vi "Check Device Out.vi"(8 "error in (no error)":errorcluster, 10 "Device GUID":string, 11 "Controller in":refnum<class "Controller.lvclass">) -> (0 "error out":errorcluster, 3 "Controller out":refnum<class "Controller.lvclass">)   [LabVIEW 2016, in "Controller Actor.lvlib" / "Controller.lvclass"]
uses:
  <userlib>/Common Components/Controller/Controller.lvclass
  <userlib>/Common Components/Controller UI/Update DT event data.ctl
  <userlib>/Common Components/Controller UI/Update DT Cmd.ctl
  <userlib>/Common Components/Controller UI/Update DT event data - checked out.ctl
  <userlib>/Common Components/Controller UI Messages/Update DT Event Msg/Update DT Event Msg.lvclass/Update DT Event Msg.ctl
  <vilib>/ActorFramework/Message Enqueuer/Message Enqueuer.lvclass/Message Enqueuer.ctl
  <vilib>/ActorFramework/Message Enqueuer/Enqueue.vi
  <userlib>/Common Components/Controller UI Messages/Update DT Event Msg/Update DT Event Msg.lvclass
  C:/Program Files (x86)/National Instruments/LabVIEW 2016/vi.lib/ActorFramework/Message/Message.lvclass
  <vilib>/ActorFramework/Message Priority Queue/Priority Enqueue.vi
  <userlib>/Common Components/Controller UI/Controller UI.lvclass
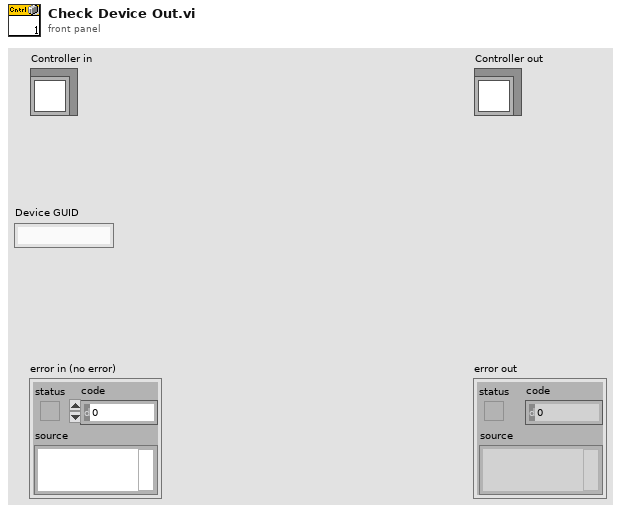
[diagram p1: front panel]
types:
  T1 = typedef "Controller UI.lvlib/Controller UI.lvclass/Update DT event data - checked out.ctl" = cluster{"GUID":string, "checked-out?":bool}
  T2 = typedef "Controller UI.lvlib/Controller UI.lvclass/Update DT event data.ctl" = cluster{"Cmd":T3, "Data Array":variant[]}
  T3 = typedef "Controller UI.lvlib/Controller UI.lvclass/Update DT Cmd.ctl" = enum16{"Update HWtype\\HWplugin array", "Update Checked-out", "Update COMM Status", "Load DevInfo from File", "Save DevInfo to File", "Update COMM Address List"}
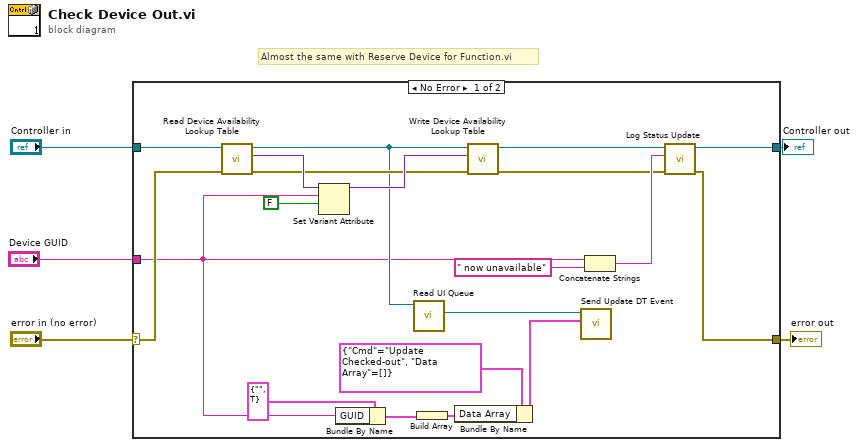
[diagram p0: block diagram]
diagram:
  # "Almost the same with Reserve Device for Function.vi"
  n1 = case shown="No Error" "error in (no error)" {
    selector: "error in (no error)" -> [w16 w27]
    tunnel: [w15 w27] -> w4
    tunnel: [w19 w26] -> w2
    tunnel: "Controller in" -> [w25 w26]
    tunnel: "Device GUID" -> [w10 _]
    frame No Error {
      n2 = call <userlib>:"Read Device Availability Lookup Table.vi"("error in (no error)"=w16, "Controller in"=w25) -> ("error out"=w18:errorcluster, "Device Availability Lookup Table"=w24:variant, "Controller out"=w14:refnum<class "Controller.lvclass">)  [unwired: 7 in]
      n3 = Set Variant Attribute(Variant=w24, name=w10, value=FALSE) -> (Variant out=w23:variant)  [unwired: 1 in, 2 out]
      n4 = Bundle By Name(cluster=T1 {"GUID"="", "checked-out?"=TRUE} ("Cluster"), "GUID"=w10) -> (w8:T1)
      n5 = call <userlib>:"Read UI Queue.vi"("UI Controller in"=w14) -> ("UI Queue"=w13:refnum<class "Message Enqueuer.lvclass">)  [unwired: 8 in, 2 out]
      n6 = Build Array(w8) -> (w7:T1[])
      n7 = Bundle By Name(cluster=T2 {"Cmd"=enum."Update Checked-out", "Data Array"=[]} ("event data"), "Data Array"=w7) -> (w11:T2)
      n8 = call <userlib>:"Write Device Availability Lookup Table.vi"("error in (no error)"=w18, "Device Availability Lookup Table"=w23, "Controller in"=w14) -> ("error out"=w17:errorcluster, "Controller out"=w20:refnum<class "Controller.lvclass">)  [unwired: 7 in]
      n9 = call <userlib>:"Send Update DT Event.vi"("event data"=w11, "Message Enqueuer"=w13) -> ()  [unwired: 8 in, 2 out]
      n10 = Concatenate Strings(w10, " now unavailable" ("string")) -> (w21:string)
      n11 = call-dynamic "Log Status Update.vi"("error in (no error)"=w17, "String"=w21, "Controller in"=w20) -> ("error out"=w15:errorcluster, "Controller out"=w19:refnum<class "Controller.lvclass">)  [unwired: 7 in]
    }
    frame Error {
    }
  }
  "error out" <- w4
  "Controller out" <- w2
